vi "Read Electrical Variables Egauge.vi"(8 "error in (no error)":errorcluster, 11 "Modbus master in":refnum<class "Modbus Master.lvclass">) -> (0 "error out":errorcluster, 3 "Modbus master out":refnum<class "Modbus Master.lvclass">)   [LabVIEW 2018]
uses:
  <vilib>/Modbus/master/Modbus Master.lvclass
panel:
  out "Setpoints":u16[](array[numeric])
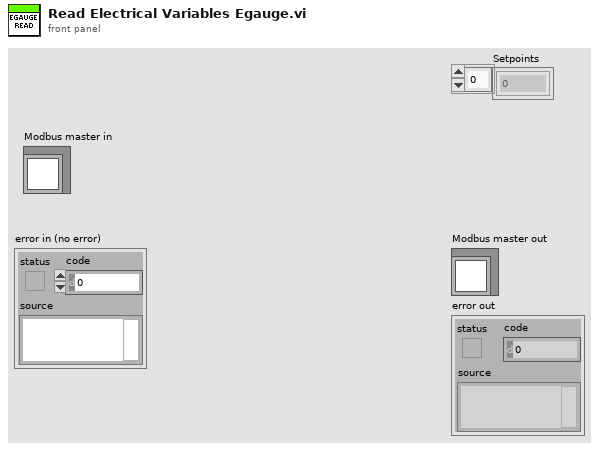
[diagram p1: front panel]
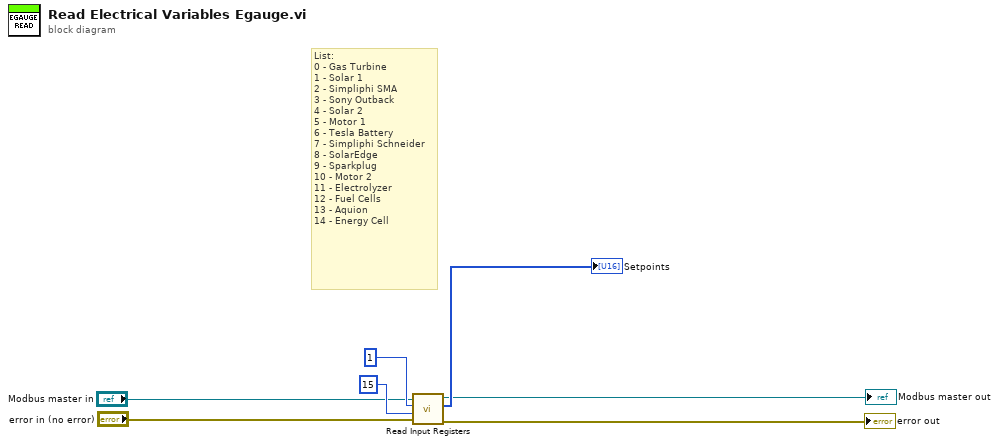
[diagram p0: block diagram]
diagram:
  # "List:\n0 - Gas Turbine\n1 - Solar 1\n2 - Simpliphi SMA\n3 - Sony Outback\n4 - Solar 2\n5 - Motor 1\n6 - Tesla Battery\n7 - Simpliphi Schneider\n8 - SolarEdge\n9 - Sparkplug\n10 - Motor 2\n11 - Electrolyzer\n12 - Fuel Cells\n13 - Aquion\n14 - Energy Cell"
  n1 = call-dynamic "Read Input Registers.vi"("error in (no error)"="error in (no error)", "number of input registers"=u16 15 ("starting address"), "starting address"=u16 1, "Modbus master in"="Modbus master in") -> ("error out"=→"error out":errorcluster, "register values"=→"Setpoints":u16[], "Modbus master out"=→"Modbus master out":refnum<class "Modbus Master.lvclass">)  [unwired: 5 in]
